vi "Logarithm.vi"(0 "argument":dbl, 5 "base":dbl, 11 "error in (no error)":errorcluster) -> (4 "exponent":dbl, 15 "error out":errorcluster)   [LabVIEW 2015]
uses:
  Exceptions/Exception Logarithm/Exception Logarithm.lvclass
  <userlib>/LV Exceptions v1/Exception/Exception.lvclass/Exception.ctl
  <vilib>/Utility/error.llb/Trim Whitespace.vi
  <userlib>/LV Exceptions v1/Exception/Exception.lvclass
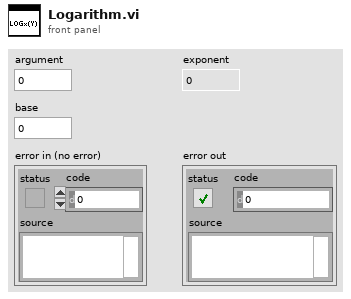
[diagram p1: front panel]
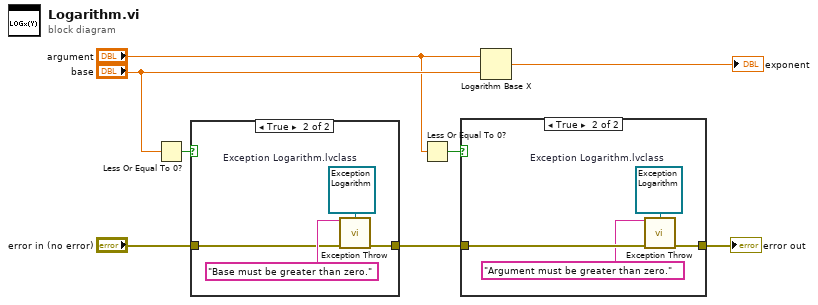
[diagram p0: block diagram]
diagram:
  n1 = Less Or Equal To 0?(x="base") -> (x <= 0?=w8:bool)
  n2 = case shown="True" w8 {
    tunnel: "error in (no error)" -> [w9 w12]
    tunnel: [w9 w11] -> w6
    frame False {
    }
    frame True {
      w10 = refnum<class "Exception Logarithm.lvclass"> refnum  # Exception Logarithm.lvclass
      n3 = call <userlib>:"Exception Throw.vi"("message"="Base must be greater than zero.", "Exception in"=w10, "error in (no error)"=w12) -> ("error out"=w11:errorcluster)  [unwired: 12 in]
    }
  }
  n4 = Less Or Equal To 0?(x="argument") -> (x <= 0?=w4:bool)
  n5 = case shown="True" w4 {
    tunnel: w6 -> [w14 w17]
    tunnel: [w14 w16] -> w5
    frame False {
    }
    frame True {
      w18 = refnum<class "Exception Logarithm.lvclass"> refnum  # Exception Logarithm.lvclass
      n6 = call <userlib>:"Exception Throw.vi"("message"="Argument must be greater than zero.", "Exception in"=w18, "error in (no error)"=w17) -> ("error out"=w16:errorcluster)  [unwired: 12 in]
    }
  }
  "error out" <- w5
  n7 = Logarithm Base X(1:"base", 2:"argument") -> (0:→"exponent":dbl)
